vi "Teleop.vi"(10 "Match Info":T1={"Autonomous Elapsed Seconds"=0.0, "TeleOp Elapsed Seconds"=0.0, "Disabled Elapsed Seconds"=0.0, "Visited Autonomous"=FALSE, "Visited TeleOp"=FALSE, "Visited Disabled"=FALSE, "Autonomous Settings"={"Autonomous Style"=enum."Independent", "VI Refnum"=refnum}}, 11 "Call Context":T2) -> ()   [LabVIEW 2011]
doc: "This VI is called for each TeleOp packet received from the DS where the robot is not disabled. It is often used to read from the joysticks and update I/O or to update setpoints for timed control loops. It should complete and return within 20 milliseconds or it may miss DS packets."
uses:
  <vilib>/Rock Robotics/WPI/DriverStation/WPI_DriverStationDerivedRobotMode.ctl
  <vilib>/Rock Robotics/WPI/DriverStation/WPI_DriverStationMatch Info.ctl
  <vilib>/Rock Robotics/WPI/Relay/WPI_RelayValue.ctl
  Robot Global Data.vi
panel:
  out "Shift Control":dbl=2.0 format="%.2f"
  in  "Left High":dbl=0.2
  in  "Right High":dbl=0.8
  in  "Left Mid":dbl=0.25
  in  "Right Mid":dbl=0.7
  in  "Shift Input 2":dbl
  in  "Left Low":dbl=0.8
  in  "Right Low":dbl=0.4
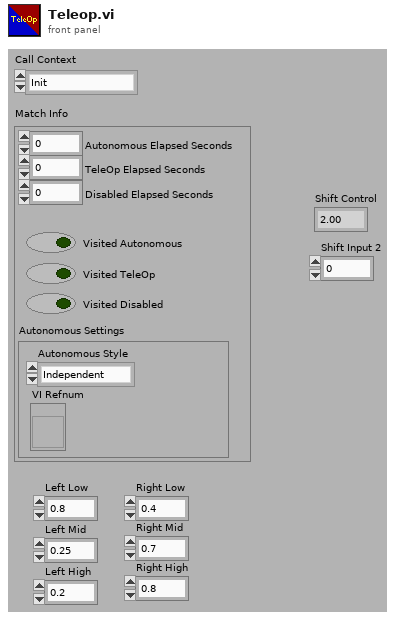
[diagram p1: front panel]
types:
  T1 = typedef "WPI_DriverStationMatch Info.ctl" = cluster{"Autonomous Elapsed Seconds":dbl, "TeleOp Elapsed Seconds":dbl, "Disabled Elapsed Seconds":dbl, "Visited Autonomous":bool, "Visited TeleOp":bool, "Visited Disabled":bool, "Autonomous Settings":cluster{"Autonomous Style":enum16{"Iterative", "Independent"}, "VI Refnum":refnum<vi>}}
  T2 = typedef "WPI_DriverStationDerivedRobotMode.ctl" = enum16{"Init", "Execute", "Stop"}
  T3 = typedef "WPI_RelayValue.ctl" = enum16{"Off", "On", "Forward", "Reverse"}
  T4 = typedef "WPI_MotorControlDeviceRef.ctl" = cluster{"DeviceStatus":errorcluster, "Type":enum16{"PWM", "CAN"}, "PWM":cluster{"Digital Module":T5, "PWM Channel":T6, "DeadBand":T7}, "CAN":cluster{"Device Number":u8, "Control Mode":T8, "Semaphore":T9, "Max Vout":dbl}, "Invert":bool, "TransformRef":T10, "InvTransformRef":T10}
  T5 = typedef "FPGA_TypedefDigitalModule.ctl" = enum16{"Digital Module 1", "Digital Module 2"}
  T6 = typedef "FPGA_DIOPWMChannel.ctl" = enum8{"PWM 1", "PWM 2", "PWM 3", "PWM 4", "PWM 5", "PWM 6", "PWM 7", "PWM 8", "PWM 9", "PWM 10", "Invalid"}
  T7 = typedef "WPI_PWMDeadband.ctl" = cluster{"Name":string, "maxPositivePwm":i32, "minPositivePwm":i32, "centerPwm":i32, "maxNegativePwm":i32, "minNegativePwm":i32, "angularRange":u16}
  T8 = typedef "WPI_CANJaguar_ControlMode.ctl" = enum8{"Percent VBus", "Current", "Speed", "Position", "Voltage"}
  T9 = typedef "Semaphore RefNum" = refnum<k1>
  T10 = typedef "WPI_PWMTransform_ConPane.ctl" = refnum<vi>
  T11 = typedef "WPI_RelayDevRef.ctl" = cluster{"DevStatus":errorcluster, "Relay Channel":T12, "Digital Module":T5, "Relay Direction":T13}
  T12 = typedef "FPGA_DIORelayChannel.ctl" = enum8{"Relay 1", "Relay 2", "Relay 3", "Relay 4", "Relay 5", "Relay 6", "Relay 7", "Relay 8", "Invalid"}
  T13 = typedef "WPI_RelayDirection.ctl" = enum16{"Both directions", "Forward only", "Reverse only"}
  T14 = typedef "WPI_ServoDeviceRef.ctl" = cluster{"DeviceStatus":errorcluster, "Digital Module":T5, "PWM Channel":T6, "DeadBand":T7}
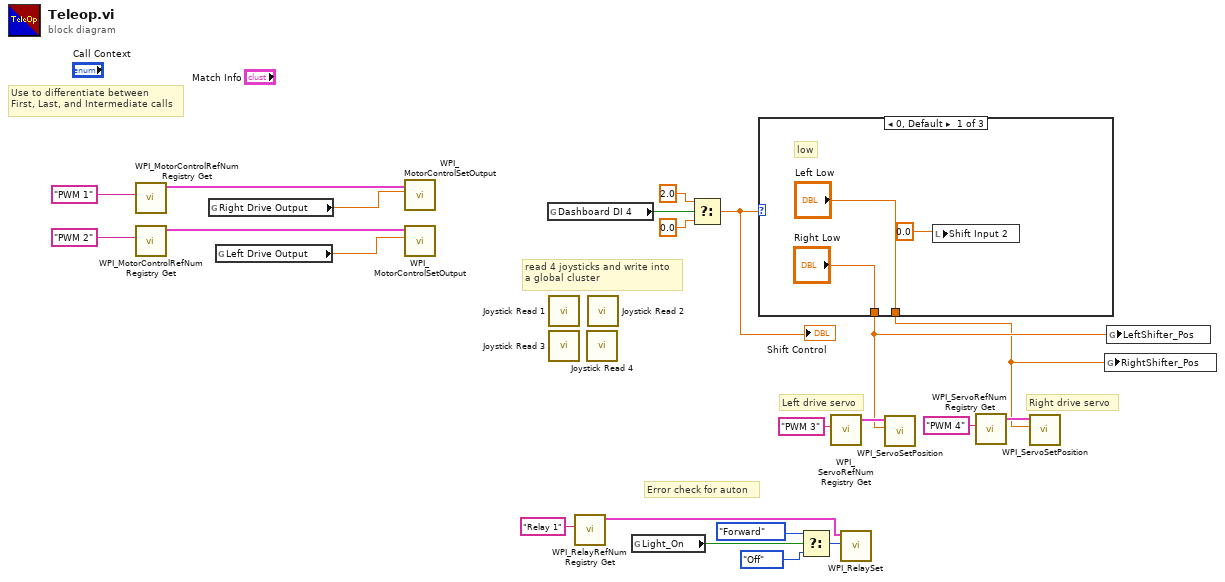
[diagram p0: block diagram]
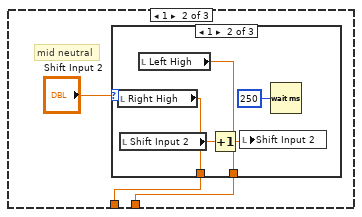
[diagram p2: hidden frame]
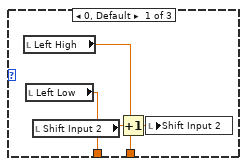
[diagram p3: hidden frame]
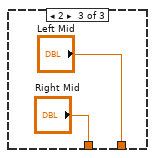
[diagram p4: hidden frame]
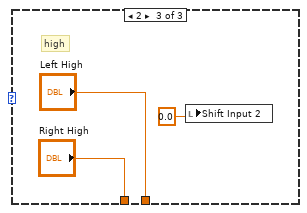
[diagram p5: hidden frame]
diagram:
  # "Error check for auton"
  # "read 4 joysticks and write into\na global cluster"
  # "Right drive servo"
  # "Left drive servo"
  # "Use to differentiate between\nFirst, Last, and Intermediate calls"
  n1 = call <vilib>:"WPI_MotorControlRefNum Registry Get.vi"("refnum name"="PWM 1") -> ("MotorControlDevRef"=w16:T4)  [unwired: 1 in, 9 out]
  n2 = call <vilib>:"WPI_MotorControlRefNum Registry Get.vi"("refnum name"="PWM 2") -> ("MotorControlDevRef"=w18:T4)  [unwired: 1 in, 9 out]
  n3 = global read "Robot Global Data.vi" "Right Drive Output"() -> (w2:dbl)
  n4 = global read "Robot Global Data.vi" "Left Drive Output"() -> (w1:dbl)
  n5 = call <vilib>:"WPI_MotorControlSetOutput.vi"("Output"=w2, "MotorControlDevRef"=w16) -> ()  [unwired: 3 in, 7 out]
  n6 = call <vilib>:"WPI_MotorControlSetOutput.vi"("Output"=w1, "MotorControlDevRef"=w18) -> ()  [unwired: 3 in, 7 out]
  n7 = global read "Robot Global Data.vi" "Dashboard DI 4"() -> (w11:bool)
  n8 = call "Joystick Read 1.vi"() -> ()  [unwired: 28 out]
  n9 = call "Joystick Read 3.vi"() -> ()  [unwired: 28 out]
  n10 = call <vilib>:"WPI_RelayRefNum Registry Get.vi"("refnum name"="Relay 1") -> ("RelayDevRef"=w5:T11)  [unwired: 1 in, 9 out]
  n11 = call "Joystick Read 4.vi"() -> ()  [unwired: 28 out]
  n12 = call "Joystick Read 2.vi"() -> ()  [unwired: 28 out]
  n13 = global read "Robot Global Data.vi" "Light_On"() -> (w4:bool)
  n14 = Select(t=2.0, s=w11, f=0.0) -> (s? t:f=w13:dbl)
  "Shift Control" <- w13
  n15 = case shown="0, Default" w13 {
    tunnel: ["Left Low" w27 "Left High"] -> w9
    tunnel: ["Right Low" w26 "Right High"] -> w10
    frame 0, Default {
      # "low"
      n16 = local write "Shift Input 2"(0.0 ("Input 2")) -> ()
    }
    frame 1 {
      # "mid neutral"
      n17 = case shown="1" "Shift Input 2" {
        tunnel: [w32 w33 "Left Mid"] -> w27
        tunnel: [w31 w34 "Right Mid"] -> w26
        frame 0, Default {
          n18 = local read "Left High"() -> (w32:dbl)
          n19 = local read "Left Low"() -> (w31:dbl)
          n20 = local read "Shift Input 2"() -> (w30:dbl)
          n21 = Increment(x=w30) -> (x+1=w29:dbl)
          n22 = local write "Shift Input 2"(w29) -> ()
        }
        frame 1 {
          n23 = local read "Right High"() -> (w34:dbl)
          n24 = local read "Shift Input 2"() -> (w36:dbl)
          n25 = local read "Left High"() -> (w33:dbl)
          n26 = Increment(x=w36) -> (x+1=w35:dbl)
          n27 = local write "Shift Input 2"(w35) -> ()
          n28 = Wait (ms)(milliseconds to wait=u32 250) -> ()  [unwired: 1 out]
        }
        frame 2 {
        }
      }
    }
    frame 2 {
      # "high"
      n29 = local write "Shift Input 2"(0.0 ("Input 2")) -> ()
    }
  }
  n30 = Select(t=WPI_RelayValue."Forward" ("RelayValue"), s=w4, f=WPI_RelayValue."Off" ("RelayValue")) -> (s? t:f=w6:T3)
  n31 = call <vilib>:"WPI_ServoRefNum Registry Get.vi"("refnum name"="PWM 3") -> ("ServoDeviceRef"=w22:T14)  [unwired: 1 in, 9 out]
  n32 = call <vilib>:"WPI_RelaySet.vi"("RelayValue"=w6, "RelayDevRef"=w5) -> ()  [unwired: 1 in, 9 out]
  n33 = call <vilib>:"WPI_ServoSetPosition.vi"("Position"=w10, "ServoDeviceRef"=w22) -> ()  [unwired: 1 in, 9 out]
  n34 = call <vilib>:"WPI_ServoRefNum Registry Get.vi"("refnum name"="PWM 4") -> ("ServoDeviceRef"=w14:T14)  [unwired: 1 in, 9 out]
  n35 = call <vilib>:"WPI_ServoSetPosition.vi"("Position"=w9, "ServoDeviceRef"=w14) -> ()  [unwired: 1 in, 9 out]
  n36 = global write "Robot Global Data.vi" "RightShifter_Pos"(w9) -> ()
  n37 = global write "Robot Global Data.vi" "LeftShifter_Pos"(w10) -> ()
